vi "Global Servo Controls.vi"() -> ()   [LabVIEW 2013]
panel:
  in  "Servo 6 (0-255)":u8=128
  in  "Servo 5 (0-255)":u8=128
  in  "Servo 4 (0-255)":u8=128
  in  "Servo 3 (0-255)":u8=128
  in  "Servo 2 (0-255)":u8=128
  in  "Servo 1 (0-255)":u8=128
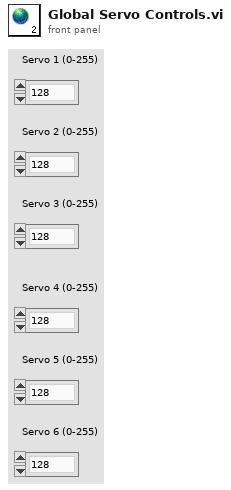
[diagram p1: front panel]
diagram:
